vi "Remove Frames.vi"(8 "error in (no error)":errorcluster, 9 "Frames":string[](array[string]), 10 "Action":T1, 11 "Custom Device reference in":refnum<k24>) -> (0 "error out":errorcluster, 3 "Custom Device reference out":refnum<k24>)   [LabVIEW 2013, in "J1939 System Definition API Support.lvlib"]
uses:
  J1939 System Definition API Support.lvlib
  NationalInstruments.VeriStand.SystemDefinitionAPI
  Types/Remove Frame Action.ctl
  Shared/SubVIs/Constants.vi
  <vilib>/NI Veristand/Custom Device Tools/Custom Device Utility Library/NI VeriStand - Search for All Items by GUID.vi
  <vilib>/NI Veristand/Custom Device Tools/Custom Device Utility Library/NI VeriStand - Search for Item by Name.vi
  <vilib>/NI Veristand/Custom Device Tools/Custom Device Utility Library/Custom Device Utility Library.lvlib
  Shared/J1939 Addon Shared.lvlib
  <vilib>/NI Veristand/Custom Device API/Custom Device API.lvlib
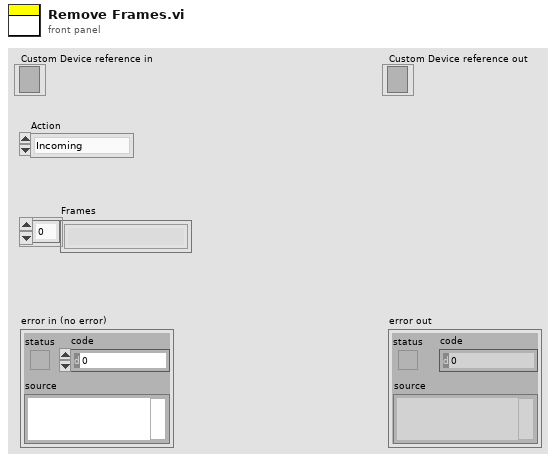
[diagram p1: front panel]
types:
  T1 = typedef "J1939 System Definition API Support.lvlib/Remove Frame Action.ctl" = enum16{"Incoming", "Outgoing"}
  T2 = typedef "Custom Device API.lvlib/Custom Device Item Ref.ctl" = u64
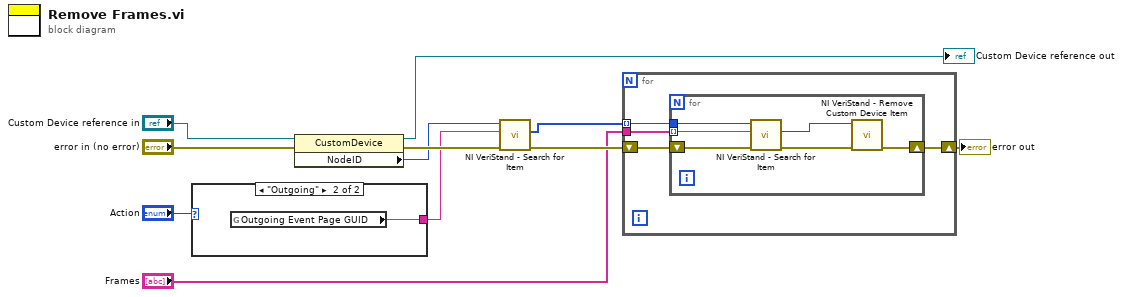
[diagram p0: block diagram]
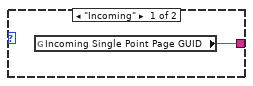
[diagram p2: hidden frame]
diagram:
  n1 = case shown="\"Outgoing\"" "Action" {
    tunnel: [w12 w13] -> w7
    frame "Incoming" {
      n2 = global read "Constants.vi" "Incoming Single Point Page GUID"() -> (w12:string)
    }
    frame "Outgoing" {
      n3 = global read "Constants.vi" "Outgoing Event Page GUID"() -> (w13:string)
    }
  }
  n4 = property class="CustomDevice"(reference="Custom Device reference in", error in="error in (no error)") -> (reference out=→"Custom Device reference out":refnum<k24>, error out=w8:errorcluster, "NodeID"=w6:u64)
  n5 = call-poly <vilib>:"NI VeriStand - Search for Item.vi"("error in"=w8, "Item GUID"=w7, "Section Ref in"=w6) -> ("error out"=w4:errorcluster, "Item Refs"=w5:T2[])  [unwired: 5 in, 2 out]
  n6 = for {
    tunnel: w5 -> [w17] mode=indexing
    tunnel: "Frames" -> [w14]
    shift-right: [w15] -> w3
    shift-left: w4 -> [w16]
    n7 = for {
      tunnel: w17 -> [w23]
      tunnel: w14 -> [w21] mode=indexing
      shift-right: [w18] -> w15
      shift-left: w16 -> [w22]
      n8 = call-poly <vilib>:"NI VeriStand - Search for Item.vi"("error in"=w22, "Item Name"=w21, "Section Ref in"=w23) -> ("error out"=w19:errorcluster, "Item Ref"=w20:T2)  [unwired: 5 in, 2 out]
      n9 = call <vilib>:"NI VeriStand - Remove Custom Device Item.vi"("error in (no error)"=w19, "Item Ref in"=w20) -> ("error out"=w18:errorcluster)  [unwired: 8 in, 1 out]
    }
  }
  "error out" <- w3
